vi "init Jl server & LV client.vi"(8 "error in (no error)":errorcluster, 11 "Julia user functions script":path) -> (0 "error out":errorcluster, 2 "Jl Server state out":T1, 3 "timeout?":bool)   [LabVIEW 2018, in "LV-0mq-Julia_roundtrip-lib.lvlib"]
doc: "Init Julia server & LabView client."
uses:
  LV-0mq-Julia_roundtrip-lib.lvlib
  Server or client state.ctl
  Commands.ctl
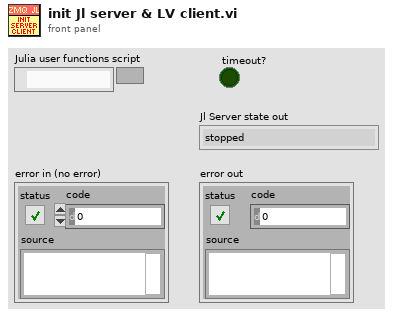
[diagram p1: front panel]
types:
  T1 = typedef "LV-0mq-Julia_roundtrip-lib.lvlib/Server or client state.ctl" = enum16{"stopped", "running", "unknown"}
  T2 = typedef "LV-0mq-Julia_roundtrip-lib.lvlib/Commands.ctl" = enum16{"Start Jl-server & Init LV-client", "Send request & Get response ", "Stop Jl-server & Cleanup LV-client", "Cleanup LV-client", "Start Jl-server", "Stop Jl-server", "Init LV-Client", "Cleanup LV-Client", "(not allowed)", "Set LV Client state", "Set Jl Server state", "set ZMQ timeout", "read ZMQ timeout", "read-out state"}
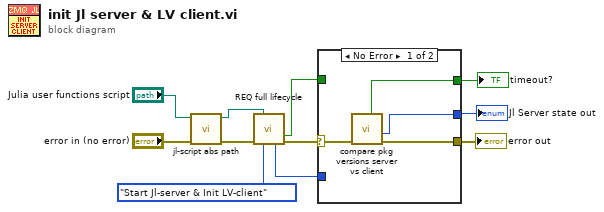
[diagram p0: block diagram]
diagram:
  n1 = call "jl-script abs path.vi"("error in (no error)"="error in (no error)", "Julia user functions script"="Julia user functions script") -> ("error out"=w3:errorcluster, "script abs path"=w2:path)  [unwired: 8 in]
  n2 = call "REQ full lifecycle.vi"("Julia user functions script"=w2, "error in"=w3, "command"=Commands."Start Jl-server & Init LV-client") -> ("timeout?"=w7:bool, "Jl Server state out"=w10:T1, "error out"=w6:errorcluster)  [unwired: 6 in, 4 out]
  n3 = case shown="No Error" w6 {
    selector: w6 -> [w15 w17]
    tunnel: [w13 w18] -> w8
    tunnel: w7 -> [_ w18]
    tunnel: [w14 w17] -> w9
    tunnel: [w12 w16] -> w11
    tunnel: w10 -> [_ w16]
    frame No Error {
      n4 = call "compare pkg versions server vs client.vi"("error in (no error)"=w15) -> ("error out"=w14:errorcluster, "Jl Server state out"=w12:T1, "timeout?"=w13:bool)  [unwired: 4 in, 4 out]
    }
    frame Error {
    }
  }
  "Jl Server state out" <- w11
  "error out" <- w9
  "timeout?" <- w8
